vi "Get Temp Setpoint Data--Accessor.vi"(8 "error in (no error)":errorcluster, 11 "Simulated Thermal Process Controller in":refnum<class "Simulated Thermal Process Controller.lvclass">) -> (0 "error out":errorcluster, 2 "Temp Setpoint Data":T1, 3 "Simulated Thermal Process Controller out":refnum<class "Simulated Thermal Process Controller.lvclass">)   [LabVIEW 2024, in "Simulated Thermal Process Controller.lvclass"]
uses:
  Simulated Thermal Process Controller.lvclass
  Process Controller/Controls/Temp Data--Cluster.ctl
  Process Controller/Controls/Temperature Units--Enum.ctl
  Simulated Thermal Process Controller.lvclass/Simulated Thermal Process Controller.ctl
  Process Controller/_Thermal Process Controller.lvclass
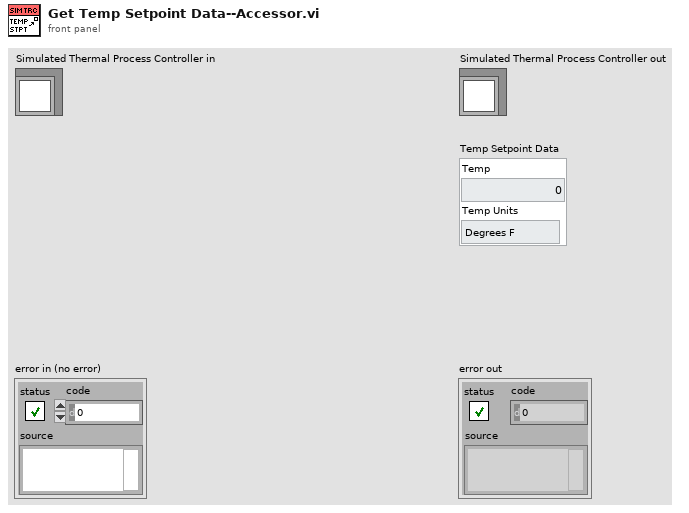
[diagram p1: front panel]
types:
  T1 = typedef "_Thermal Process Controller.lvclass/Temp Data--Cluster.ctl" = cluster{"Temp":dbl, "Temp Units":T2}
  T2 = typedef "_Thermal Process Controller.lvclass/Temperature Units--Enum.ctl" = enum16{"Degrees F", "Degrees C", "Degrees K"}
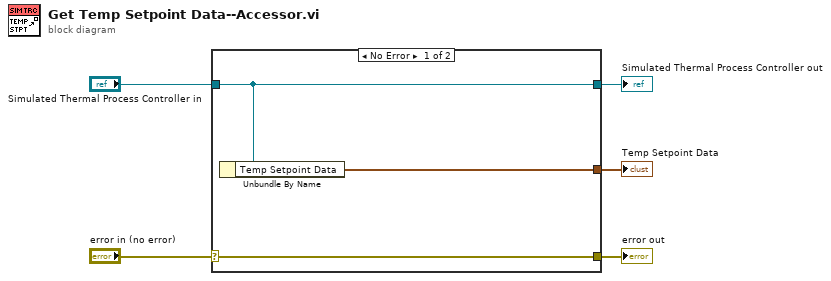
[diagram p0: block diagram]
diagram:
  n1 = case shown="No Error" "error in (no error)" {
    selector: "error in (no error)" -> [w8 w9]
    tunnel: [w8 w9] -> w4
    tunnel: [w7 w10] -> w2
    tunnel: "Simulated Thermal Process Controller in" -> [w7 w10]
    tunnel: [w6 _] -> w1
    frame No Error {
      n2 = Unbundle By Name(w7) -> ("Temp Setpoint Data"=w6:T1)
    }
    frame Error {
    }
  }
  "error out" <- w4
  "Simulated Thermal Process Controller out" <- w2
  "Temp Setpoint Data" <- w1
